vi "AlliGator FMB Save Simulation Results (1).vi"(7 "File Path (Dialog if empty)":path, 8 "error in (no error)":errorcluster, 9 "Fit Settings":T15 {"Decay Fit Options"."Confidence Level" min=0.0 max=100.0; "Decay Fit Options"."Offset Resolution" min=0.0; "Decay Fit Options"."Period" min=0.0; "Decay Fit Options"."Min Decay Percentile" min=0.0 max=1.0; "Decay Fit Options"."Max Decay Percentile" min=0.0 max=100.0; "Fit Parameter Constraints"."Max Value" format="%#.3g"; "Fit Parameter Constraints"."Min Value" format="%#.3g"}, 10 "Simulation Parameters":T2={"Decay Simulation Parameters"={"tau 1"=1e-09, "tau 2"=0.0, "a1"=1.0, "Baseline"=0.0}, "Fit Simulation Parameters"={"# Counts"=100, "# Simulations (N)"=100, "Decay Bin Size"=1.0000000000000002e-10, "# Bins"=200}, "Use Experimental IRF"=FALSE}, 11 "Fit Results":cluster{"Fit Results":T1[]}) -> (0 "error out":errorcluster, 3 "Message":string)   [LabVIEW 2021, in "AlliGator Fit Method Benchmark.lvlib"]
uses:
  AlliGator Fit Method Benchmark.lvlib
  Fits/IRF(X)PSED/Decay Fit Options v4.ctl
  Fits/Decay Convolution/Decay Model.ctl
  Fits/Residual Type.ctl
  Fits/IRF(X)PSED/Fit Weights Type v2.ctl
  Fits/Non-linear Fitting Method v2.ctl
  Fits/Fit Calculation Method.ctl
  Fits/Non-linear Fitting Algorithm.ctl
  Decay Analysis/Decay Fit/AlliGator Decay Fit Parameter Constraints 2.ctl
  Fits/IRF(X)PSED/Decay Fit Parameters In List.ctl
  Fits/IRF(X)PSED/MLE Baseline Offset Type.ctl
  AlliGator Simulation Parameters.ctl
  AlliGator Decay Simulation Parameters.ctl
  AlliGator Fit Simulation Parameters.ctl
  Fits/IRF(X)PSED/IRF(X)PSED Fit Results.ctl
  Fits/IRF(X)PSED/Decay Fit Parameters & Derived Quantities List v2.ctl
  <vilib>/Utility/file.llb/Write Delimited Spreadsheet (DBL).vi
  Fits/Fits.lvlib
  Variant/Variant.lvlib
  Files/Files.lvlib
  Decay Analysis/Decay Fit/AlliGator Decay Fit.lvlib
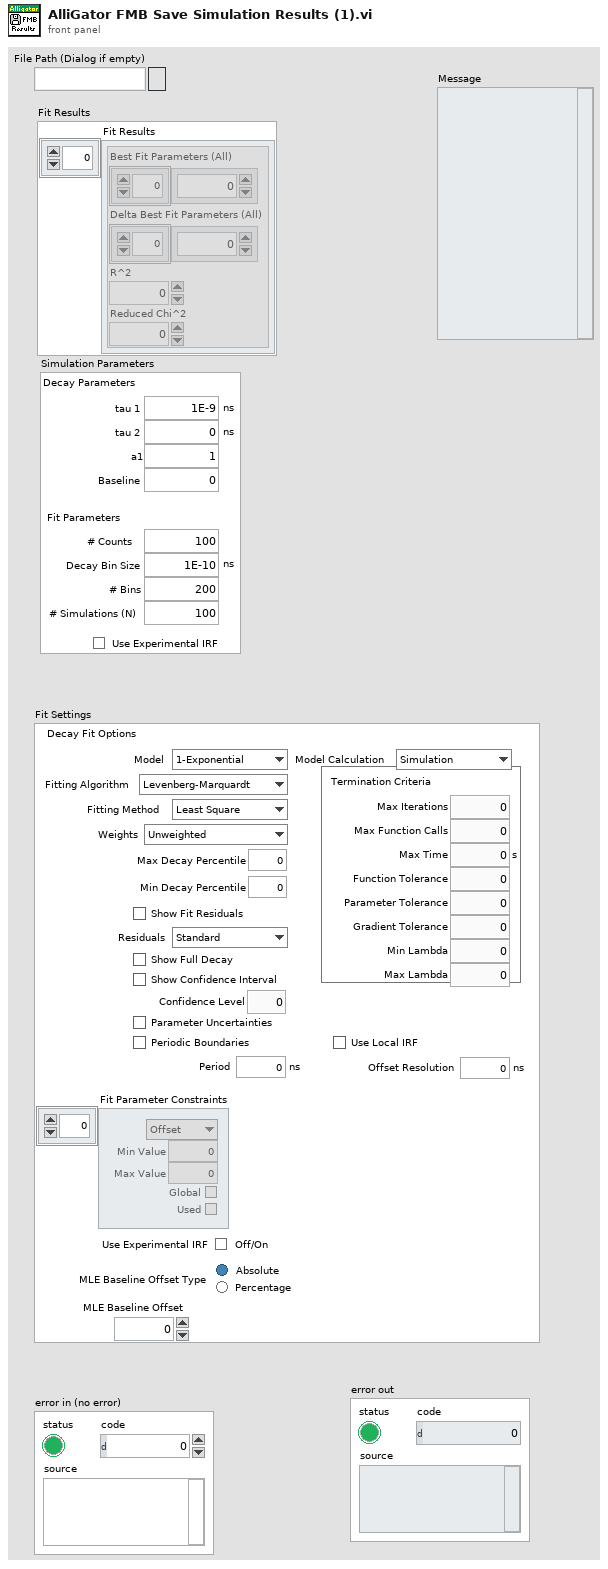
[diagram p1: front panel]
types:
  T1 = typedef "Fits.lvlib/IRF(X)PSED Fit Results.ctl" = cluster{"Best Fit Parameters (All)":dbl[], "Delta Best Fit Parameters (All)":dbl[], "R^2":dbl, "Reduced Chi^2":dbl}
  T2 = typedef "AlliGator Fit Method Benchmark.lvlib/AlliGator Simulation Parameters.ctl" = cluster{"Decay Simulation Parameters":T3, "Fit Simulation Parameters":T4, "Use Experimental IRF":bool}
  T3 = typedef "AlliGator Fit Method Benchmark.lvlib/AlliGator Decay Simulation Parameters.ctl" = cluster{"tau 1":dbl[unit], "tau 2":dbl[unit], "a1":dbl, "Baseline":dbl}
  T4 = typedef "AlliGator Fit Method Benchmark.lvlib/AlliGator Fit Simulation Parameters.ctl" = cluster{"# Counts":i32, "# Simulations (N)":i32, "Decay Bin Size":dbl[unit], "# Bins":i32}
  T5 = typedef "Fits.lvlib/Decay Fit Options v4.ctl" = cluster{"Show Fit Residuals":bool, "Fit Model":T6, "Residual Type":T7, "Max Decay Percentile":dbl, "Min Decay Percentile":dbl, "Show Full Decay":bool, "Weights":T8, "Fitting Method":T9, "Compute Parameter Uncertainties":bool, "Periodic Boundaries":bool, "Model Calculation":T10, "Period":dbl[unit], "Termination Criteria":cluster{"Max Iterations":i32, "Max Function Calls":i32, "Max Time":dbl[unit], "Function Tolerance":dbl, "Parameter Tolerance":dbl, "Gradient Tolerance":dbl, "Min Lambda":dbl, "Max Lambda":dbl, "Initial Tick Count":u32}, "Offset Resolution":dbl[unit], "Use Local IRF":bool, "Fitting Algorithm":T11, "Show Confidence Interval ":bool, "Confidence Level":dbl}
  T6 = typedef "Fits.lvlib/Decay Model.ctl" = enum16{"1-Exponential", "2-Exponentials"}
  T7 = typedef "Fits.lvlib/Residual Type.ctl" = enum16{"Standard", "Normalized", "Reduced"}
  T8 = typedef "Fits.lvlib/Fit Weights Type v2.ctl" = enum16{"Unweighted", "1/Variance (Neyman)", "1/Variance (Pearson)", "Best of All"}
  T9 = typedef "Fits.lvlib/Non-linear Fitting Method v2.ctl" = enum16{"Least Square", "Least Absolute Residual", "Bisquare", "MLE", "-", "Best of All"}
  T10 = typedef "Fits.lvlib/Fit Calculation Method.ctl" = enum16{"Simulation", "Convolution", "Integration"}
  T11 = typedef "Fits.lvlib/Non-linear Fitting Algorithm.ctl" = enum16{"Levenberg-Marquardt", "Trust-Region Dogleg"}
  T12 = typedef "AlliGator Decay Fit.lvlib/AlliGator Decay Fit Parameter Constraints 2.ctl" = cluster{"Fit Parameter":T13, "Min Value":dbl, "Max Value":dbl, "Global":bool, "Used":bool}
  T13 = typedef "Fits.lvlib/Decay Fit Parameters In List.ctl" = enum16{"Offset", "Baseline", "A_1", "tau_1", "A_2", "tau_2"}
  T14 = typedef "Fits.lvlib/MLE Baseline Offset Type.ctl" = enum32{"Absolute", "Percentage"}
  T15 = cluster{"Decay Fit Options":T5, "Fit Parameter Constraints":T12[], "Use Experimental IRF":bool, "MLE Baseline Offset Type":T14, "MLE Baseline Offset":dbl}
  T16 = typedef "Fits.lvlib/Decay Fit Parameters & Derived Quantities List v2.ctl" = enum16{"Offset", "Baseline", "A_1", "tau_1", "A_2", "tau_2", "<tau>_a", "f1_a", "f2_a", "<tau>_i", "f1_i", "f2_i", "-", "R^2", "Chi^2"}
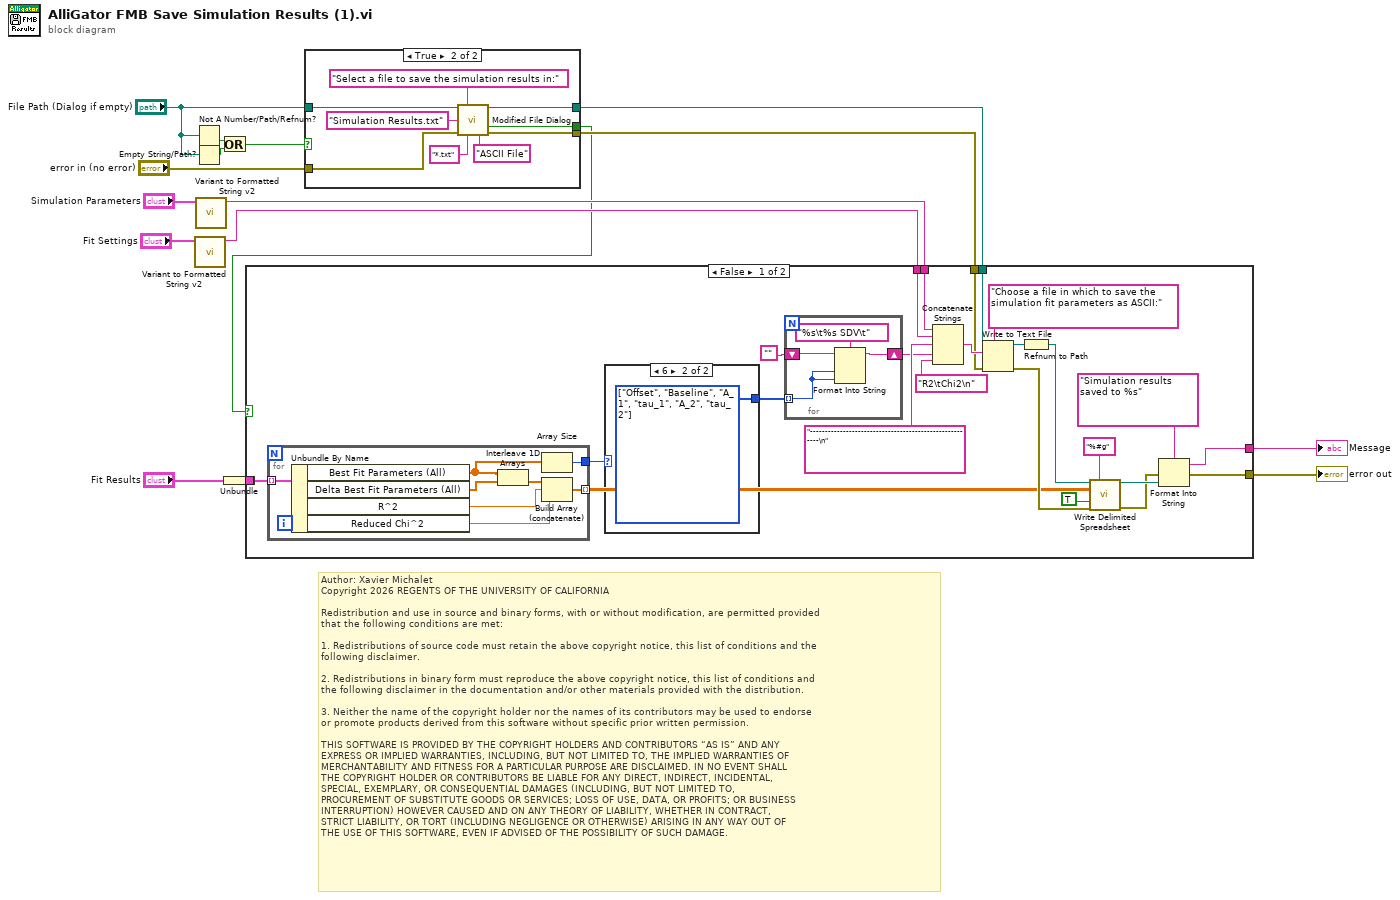
[diagram p0: block diagram]
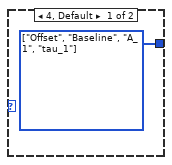
[diagram p2: hidden frame]
diagram:
  # "Author: Xavier Michalet\nCopyright 2026 REGENTS OF THE UNIVERSITY OF CALIFORNIA\n\nRedistribution and use in source and binary forms, with or without modification, are permitted provided\nthat the following conditions are met:\n\n1. Redistributions of source code must retain the above copyright notice, this list of conditions and the\nfollowing disclaimer.\n\n2. Redistributions in binary form must reproduce the above copyright notice, this list of conditions and\nthe following disclaimer in the documentation and/or other materials provided with the distribution.\n\n3. Neither the name of the copyright holder nor the names of its contributors may be used to endorse \nor promote products derived from this software without specific prior written permission.\n\nTHIS SOFTWARE IS PROVIDED BY THE COPYRIGHT HOLDERS AND CONTRIBUTORS “AS IS” AND ANY \nEXPRESS OR IMPLIED WARRANTIES, INCLUDING, BUT NOT LIMITED TO, THE IMPLIED WARRANTIES OF\nMERCHANTABILITY AND FITNESS FOR A PARTICULAR PURPOSE ARE DISCLAIMED. IN NO EVENT SHALL\nTHE COPYRIGHT HOLDER OR CONTRIBUTORS BE LIABLE FOR ANY DIRECT, INDIRECT, INCIDENTAL, \nSPECIAL, EXEMPLARY, OR CONSEQUENTIAL DAMAGES (INCLUDING, BUT NOT LIMITED TO, \nPROCUREMENT OF SUBSTITUTE GOODS OR SERVICES; LOSS OF USE, DATA, OR PROFITS; OR BUSINESS\nINTERRUPTION) HOWEVER CAUSED AND ON ANY THEORY OF LIABILITY, WHETHER IN CONTRACT, \nSTRICT LIABILITY, OR TORT (INCLUDING NEGLIGENCE OR OTHERWISE) ARISING IN ANY WAY OUT OF\nTHE USE OF THIS SOFTWARE, EVEN IF ADVISED OF THE POSSIBILITY OF SUCH DAMAGE."
  n1 = Not A Number/Path/Refnum?(number/path/refnum="File Path (Dialog if empty)") -> (NaN/Path/Refnum?=w8:bool)
  n2 = Empty String/Path?(string/path="File Path (Dialog if empty)") -> (empty?=w7:bool)
  n3 = call "Variant to Formatted String v2.vi"("Anything"="Fit Settings") -> ("String"=w15:string)  [unwired: 9 in, 1 out]
  n4 = call "Variant to Formatted String v2.vi"("Anything"="Simulation Parameters") -> ("String"=w14:string)  [unwired: 9 in, 1 out]
  n5 = Or(x=w8, y=w7) -> (x .or. y?=w6:bool)
  n6 = case shown="True" w6 {
    tunnel: "File Path (Dialog if empty)" -> [w17 w26]
    tunnel: [w17 w19] -> w4
    tunnel: "error in (no error)" -> [w16 w24]
    tunnel: [w16 w20] -> w2
    tunnel: [_ w18] -> w1
    frame False {
    }
    frame True {
      n7 = call "Modified File Dialog.vi"("Start Path"=w26, "Prompt"="Select a file to save the simulation results in:", "Suggested Filename"="Simulation Results.txt", "error in (no error)"=w24, "Pattern"="*.txt", "Pattern Label"="ASCII File") -> ("Selected Path"=w19:path, "Cancelled"=w18:bool, "error out"=w20:errorcluster)  [unwired: 6 in, 1 out]
    }
  }
  n8 = case shown="False" w1 {
    tunnel: w15 -> [w50 _]
    tunnel: w14 -> [w49 _]
    tunnel: [w46 _] -> w12
    tunnel: [w45 w66] -> w11
    tunnel: "Fit Results" -> [w29 _]
    tunnel: w4 -> [w28 _]
    tunnel: w2 -> [w27 w66]
    frame False {
      n9 = Unbundle(w29) -> ("Fit Results"=w48:T1[])
      n10 = for {
        tunnel: w48 -> [w65] mode=indexing
        tunnel: [w60] -> w30 mode=indexing
        tunnel: [w58] -> w31
        n11 = Unbundle By Name(w65) -> ("Best Fit Parameters (All)"=w59:dbl[], "Delta Best Fit Parameters (All)"=w64:dbl[], "R^2"=w62:dbl, "Reduced Chi^2"=w61:dbl)
        n12 = Interleave 1D Arrays(w59, w64) -> (w63:dbl[])
        n13 = Array Size(array=w59) -> (size(s)=w58:i32)
        n14 = Build Array (concatenate)(w63, w62, w61) -> (w60:dbl[])
      }
      n15 = case shown="6" w31 {
        tunnel: [w56 w57] -> w33
        frame 4, Default {
          w56 = T16[] [enum."Offset", enum."Baseline", enum."A_1", enum."tau_1"] items=["Offset", "Baseline", "A_1", "tau_1", "A_2", "tau_2", "<tau>_a", "f1_a", "f2_a", "<tau>_i", "f1_i", "f2_i", "-", "R^2", "Chi^2"] ("Array")
        }
        frame 6 {
          w57 = T16[] [enum."Offset", enum."Baseline", enum."A_1", enum."tau_1", enum."A_2", enum."tau_2"] items=["Offset", "Baseline", "A_1", "tau_1", "A_2", "tau_2", "<tau>_a", "f1_a", "f2_a", "<tau>_i", "f1_i", "f2_i", "-", "R^2", "Chi^2"] ("Array")
        }
      }
      n16 = for {
        shift-right: [w53] -> w34
        shift-left: "" -> [w55]
        tunnel: w33 -> [w52] mode=indexing
        n17 = Format Into String(format string="%s\t%s SDV\t", initial string=w55, w52, w52) -> (resulting string=w53:string)  [unwired: 1 in, 1 out]
      }
      n18 = Concatenate Strings(w49, w50, "-------------------------------------------------------\n" ("string"), w34, "R2\tChi2\n" ("format string")) -> (w36:string)
      n19 = Write to Text File(prompt (Choose or enter file path)="Choose a file in which to save the simulation fit parameters as ASCII:", file (use dialog)=w28, text=w36, error in=w27) -> (refnum out=w38:refnum<file>, error out=w40:errorcluster)  [unwired: 1 out]
      n20 = Refnum to Path(1:w38) -> (0:w39:path)
      n21 = call-poly <vilib>:"Write Delimited Spreadsheet.vi"("file path (dialog if empty)"=w39, "format (%.3f)"="%#g", "2D data"=w30, "append to file? (new file:F)"=TRUE ("transpose? (no:F)"), "error in (no error)"=w40) -> ("new file path (Not A Path if cancelled)"=w44:path, "error out"=w43:errorcluster)  [unwired: 9 in]
      n22 = Format Into String(format string="Simulation results saved to %s", error in=w43, w44) -> (resulting string=w46:string, error out=w45:errorcluster)  [unwired: 1 in]
    }
    frame True {
    }
  }
  "Message" <- w12
  "error out" <- w11
